vi "Sender.vi"(8 "error in (no error)":errorcluster caption="错误输入（无错误）", 9 "Sender Name":string, 10 "Sender Address":string, 11 "Email In":refnum<class "Email.lvclass"> caption="DNL_LabVIEW Object in") -> (0 "error out":errorcluster caption="错误输出", 3 "Email Out":refnum<class "Email.lvclass"> caption="DNL_LabVIEW Object out")   [LabVIEW 2012, in "Email.lvclass"]
uses:
  Email.lvclass
  Email.lvclass/Email.ctl
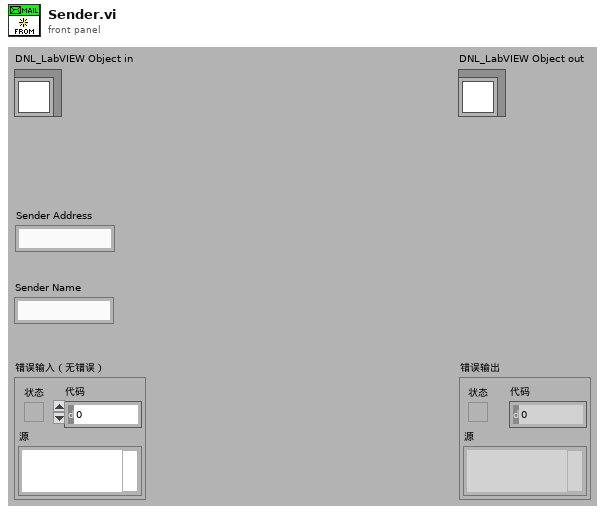
[diagram p1: front panel]
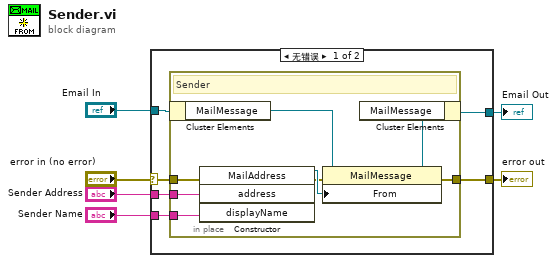
[diagram p0: block diagram]
diagram:
  n1 = case shown="无错误" "error in (no error)" {
    selector: "error in (no error)" -> [w10 w22]
    tunnel: [w7 w22] -> w5
    tunnel: [w11 w21] -> w3
    tunnel: "Email In" -> [w12 w21]
    tunnel: "Sender Address" -> [w9 _]
    tunnel: "Sender Name" -> [w8 _]
    frame No Error {
      n2 = in-place {
        in-place-border: w10 -> [w16]
        in-place-border: w9 -> [w15]
        in-place-border: w8 -> [w14]
        in-place-border: [w13] -> w7
        # "Sender"
        n3 = in-place-cluster #1(w12) -> ("MailMessage"=w20:refnum<k24>)
        n4 = constructor class="MailAddress"(error in=w16, "address"=w15, "displayName"=w14) -> (reference out=w19:refnum<k24>, error out=w18:errorcluster)  [unwired: 2 in, 3 out]
        n5 = property class="MailMessage"(reference=w20, error in=w18, "From"=w19) -> (reference out=w17:refnum<k24>, error out=w13:errorcluster)
        n6 = in-place-cluster #1("MailMessage"=w17) -> (w11:refnum<class "Email.lvclass">)
      }
    }
    frame Error {
    }
  }
  "error out" <- w5
  "Email Out" <- w3
